vi "Render Captain Part.vi"(4 "Scale":sgl, 7 "index":i32, 8 "Captain Origin":refnum<class "Vector 2D.lvclass">, 9 "Captain Hotspots":refnum<class "Vector 2D.lvclass">[](array[class]), 10 "Captain":string[](array[string]), 11 "Renderer in":refnum<class "Renderer.lvclass">) -> ()   [LabVIEW 2021, in "Ship.lvclass"]
uses:
  Ship.lvclass
  Re-use Libraries/Vector 2D/Vector 2D.lvclass
  Renderer/Renderer.lvclass
  Re-use Libraries/Vector 2D/Vector 2D.lvclass/Vector 2D.ctl
  Renderer/Renderer.lvclass/Renderer.ctl
  Texture/Texture.lvclass/Texture.ctl
  Resource Manager/Resource Manager.lvclass
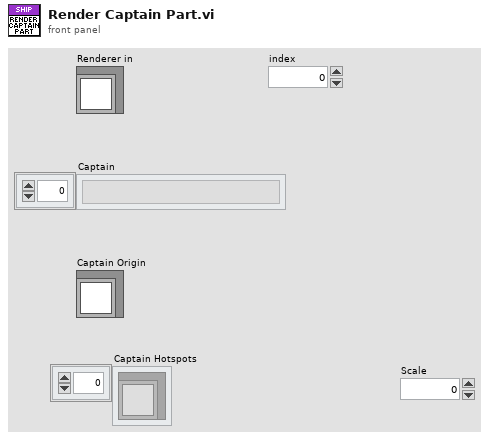
[diagram p1: front panel]
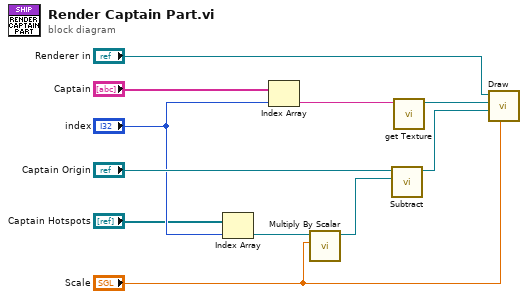
[diagram p0: block diagram]
diagram:
  n1 = Index Array(array="Captain Hotspots", index="index") -> (element=w3:refnum<class "Vector 2D.lvclass">)
  n2 = Index Array(array="Captain", index="index") -> (element=w8:string)
  n3 = call "Multiply By Scalar.vi"("x"="Scale", "A"=w3) -> ("Ax"=w2:refnum<class "Vector 2D.lvclass">)  [unwired: 9 in]
  n4 = call "Subtract.vi"("B"=w2, "A"="Captain Origin") -> ("A-B"=w9:refnum<class "Vector 2D.lvclass">)  [unwired: 9 in]
  n5 = call "get Texture.vi"("Texture Name"=w8) -> ("Texture"=w7:refnum<class "Texture.lvclass">)  [unwired: 10 in]
  n6 = call "Draw.vi"("Scale"="Scale", "Destination"=w9, "Texture"=w7, "Renderer"="Renderer in") -> ()  [unwired: 7 in, 1 out]
